vi "test.vi"() -> ()   [LabVIEW 2011, in "双模温度计2.xctl"]
panel:
  in  "双模温度计":dbl(xcontrol)
  in  "双模温度计2 2":dbl
  out "双模温度计2":dbl(xcontrol)
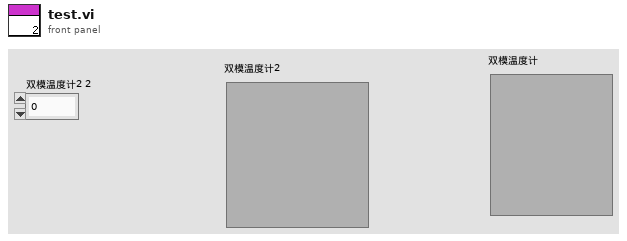
[diagram p1: front panel]
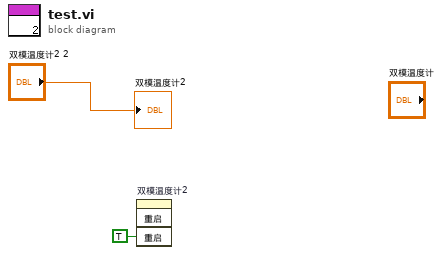
[diagram p0: block diagram]
diagram:
  n1 = invoke on="双模温度计2" class="双模温度计2 (strict)" method="重启"("重启"=TRUE) -> ()  [unwired: 3 in, 4 out]
  "双模温度计2" <- "双模温度计2 2"
